vi "zadanie3_subvi.vi"(8 "error in (no error)":errorcluster, 9 "Dalej":bool, 10 "Podaj login: in":string, 11 "Podaj hasło: in":string) -> (0 "error out":errorcluster, 1 "Podaj login: out":string, 2 "Dzisiejsza data:":string, 3 "Obecna godzina:":string, 5 "Podaj hasło: out":string)   [LabVIEW 2012]
panel:
  # "Zaloguj się aby kontynuować"
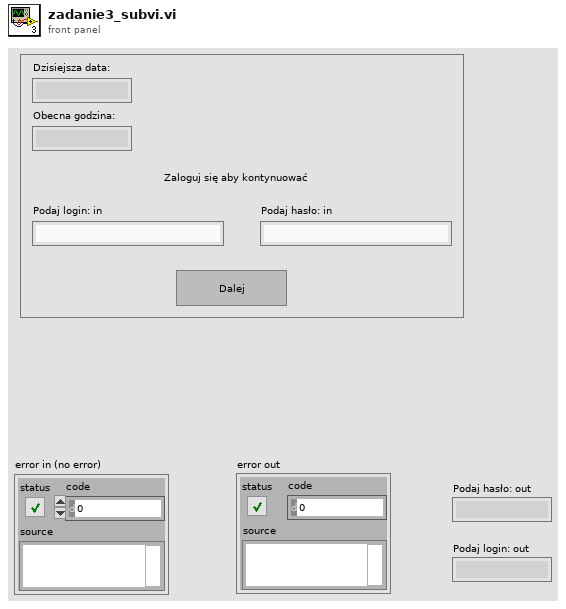
[diagram p1: front panel]
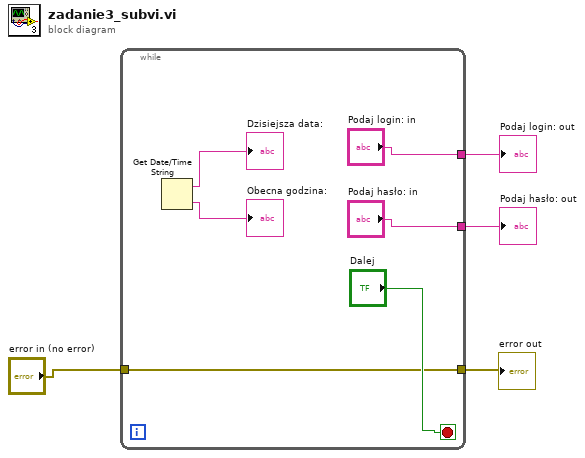
[diagram p0: block diagram]
diagram:
  n1 = while {
    tunnel: [w5] -> w2
    tunnel: ["Podaj hasło: in"] -> w3
    tunnel: ["Podaj login: in"] -> w4
    tunnel: "error in (no error)" -> [w5]
    stop <- "Dalej" stop-if-true
    n2 = Get Date/Time String() -> (date string=→"Dzisiejsza data:":string, time string=→"Obecna godzina:":string)  [unwired: 3 in]
  }
  "Podaj login: out" <- w4
  "Podaj hasło: out" <- w3
  "error out" <- w2
